vi "DWordToHex.vi"(11 "DWORD":i32[](array[numeric])) -> (3 "数组":u16[](array[numeric]) format="%04xH")   [LabVIEW 2016, in "质控单元V1.lvlib"]
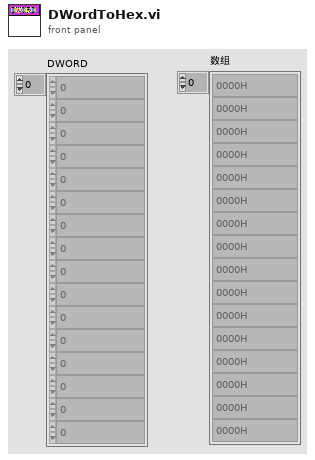
[diagram p1: front panel]
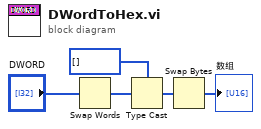
[diagram p0: block diagram]
diagram:
  n1 = Swap Words(1:"DWORD") -> (0:w1:i32[])
  n2 = Type Cast(type=u16[] [], x=w1) -> (*(type *) &x=w4:u16[])
  n3 = Swap Bytes(anything=w4) -> (byte swapped=→"数组":u16[])
